vi "Query Chain.vi"(5 "Caller Enqueuer":refnum<class "Message Enqueuer.lvclass">, 7 "Close Connections (F)":bool, 8 "error in (no error)":errorcluster, 9 "Execute IL Action (T)":bool=TRUE, 11 "Interlock Chain":refnum<class "Interlock Chain.lvclass">) -> (0 "error out":errorcluster, 1 "Interlock?":bool, 2 "Interlock out":refnum<class "Interlock.lvclass">, 3 "Interlock Chain":refnum<class "Interlock Chain.lvclass">, 4 "Stop Self?":bool, 6 "IL Action":refnum<class "IL Action.lvclass">[](array[class]))   [LabVIEW 2015, in "Interlocks.lvlib" / "Interlock Chain.lvclass"]
uses:
  Interlock Chain/Interlock Chain.lvclass
  Interlock.lvclass
  IL Action/IL Action.lvclass
  <vilib>/ActorFramework/Message Enqueuer/Message Enqueuer.lvclass
  Interlock Chain/Interlock Chain.lvclass/Interlock Chain.ctl
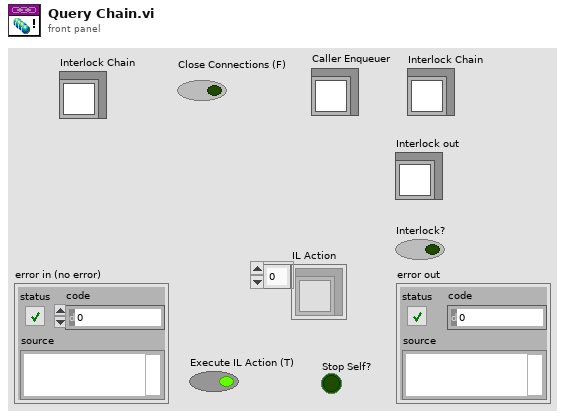
[diagram p1: front panel]
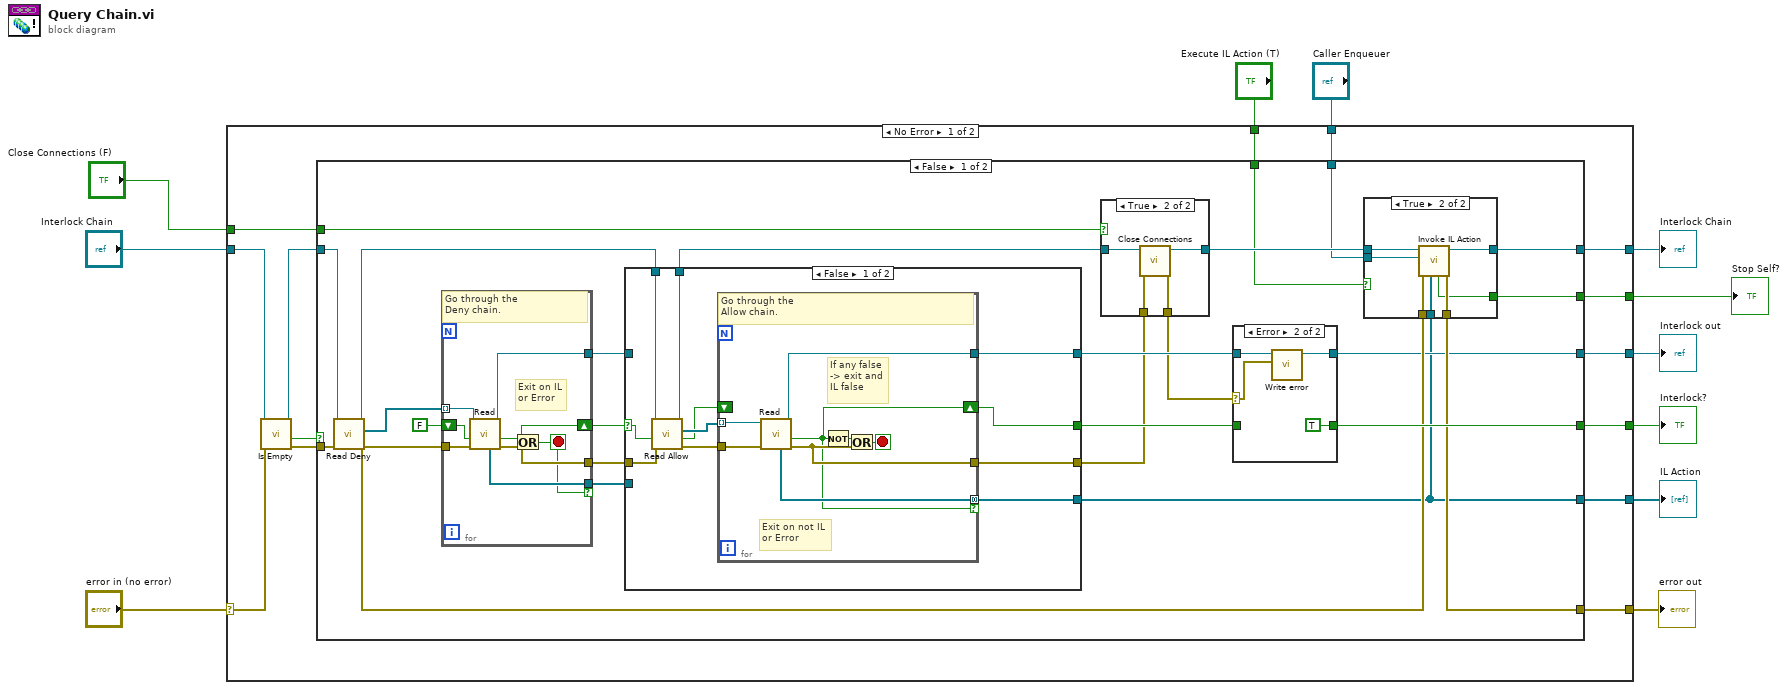
[diagram p0: block diagram]
diagram:
  n1 = case shown="No Error" "error in (no error)" {
    selector: "error in (no error)" -> [w15 w106]
    tunnel: "Interlock Chain" -> [w20 w107]
    tunnel: [w25 _] -> w11
    tunnel: [w24 _] -> w10
    tunnel: [w23 w107] -> w7
    tunnel: "Close Connections (F)" -> [w22 _]
    tunnel: [w17 _] -> w5
    tunnel: [w16 w106] -> w4
    tunnel: "Caller Enqueuer" -> [w14 _]
    tunnel: "Execute IL Action (T)" -> [w13 _]
    tunnel: [w12 _] -> w1
    frame No Error {
      n2 = call "Is Empty.vi"("error in (no error)"=w15, "Interlock Chain in"=w20) -> ("error out"=w21:errorcluster, "Is Empty?"=w18:bool, "Interlock Chain out"=w19:refnum<class "Interlock Chain.lvclass">)  [unwired: 7 in]
      n3 = case shown="False" w18 {
        tunnel: [w30 _] -> w25
        tunnel: [w41 _] -> w24
        tunnel: [w33 w105] -> w23
        tunnel: w22 -> [w39 _]
        tunnel: w21 -> [w38 w104]
        tunnel: w19 -> [w37 w105]
        tunnel: [w28 _] -> w17
        tunnel: [w31 w104] -> w16
        tunnel: w14 -> [w29 _]
        tunnel: w13 -> [w27 _]
        tunnel: [w26 _] -> w12
        frame False {
          n4 = call "Read Deny.vi"("error in (no error)"=w38, "Interlock Chain in"=w37) -> ("error out"=w32:errorcluster, "Deny"=w49:refnum<class "Interlock.lvclass">[], "Interlock Chain out"=w48:refnum<class "Interlock Chain.lvclass">)  [unwired: 7 in]
          n5 = for {
            shift-right: [w100] -> w43
            shift-left: FALSE ("Interlock out") -> [w102]
            tunnel: [w101] -> w45
            tunnel: w32 -> [w103]
            tunnel: [w98] -> w44
            tunnel: w49 -> [w99] mode=indexing
            tunnel: [w97] -> w36 if=w96
            stop <- w96 stop-if-true
            # "Exit on IL\nor Error"
            # "Go through the\nDeny chain."
            n6 = call-dynamic "Read.vi"("error in (no error)"=w103, 9:"Interlock in"=w102, 11:"Interlock in"=w99) -> ("error out"=w98:errorcluster, 1:"Interlock out"=w100:bool, 3:"Interlock out"=w101:refnum<class "Interlock.lvclass">, "IL Action"=w97:refnum<class "IL Action.lvclass">[])  [unwired: 4 in, 1 out]
            n7 = Or(x=w100, y=w98) -> (x .or. y?=w96:bool)
          }
          n8 = case shown="False" w43 {
            selector: w43 -> [w68 w89]
            tunnel: w48 -> [w76 w86]
            tunnel: [w75 w86] -> w47
            tunnel: [w70 w88] -> w46
            tunnel: w45 -> [_ w88]
            tunnel: [w69 w89] -> w42
            tunnel: [w72 w87] -> w40
            tunnel: w44 -> [w71 w87]
            tunnel: w36 -> [_ w85]
            tunnel: [w66 w85] -> w28
            frame False {
              n9 = call "Read Allow.vi"("error in (no error)"=w71, "Interlock in (False)"=w68, "Interlock Chain in"=w76) -> ("error out"=w74:errorcluster, "Interlock out"=w67:bool, "Allow"=w73:refnum<class "Interlock.lvclass">[], "Interlock Chain out"=w75:refnum<class "Interlock Chain.lvclass">)  [unwired: 5 in]
              n10 = for {
                tunnel: w74 -> [w84]
                tunnel: [w82] -> w72
                tunnel: w73 -> [w83] mode=indexing
                tunnel: [w81] -> w70
                shift-right: [w77] -> w69
                shift-left: w67 -> [_]
                tunnel: [w80] -> w66 mode=concatenating if=w77
                stop <- w79 stop-if-true
                # "If any false\n-> exit and\nIL false"
                # "Exit on not IL\nor Error"
                # "Go through the\nAllow chain."
                n11 = call-dynamic "Read.vi"("error in (no error)"=w84, "Interlock in"=w83) -> ("error out"=w82:errorcluster, 1:"Interlock out"=w77:bool, 3:"Interlock out"=w81:refnum<class "Interlock.lvclass">, "IL Action"=w80:refnum<class "IL Action.lvclass">[])  [unwired: 5 in, 1 out]
                n12 = Not(x=w77) -> (.not. x?=w78:bool)
                n13 = Or(x=w78, y=w82) -> (x .or. y?=w79:bool)
              }
            }
            frame True {
            }
          }
          n14 = case shown="True" w39 {
            tunnel: w47 -> [w61 w65]
            tunnel: [w61 w64] -> w34
            tunnel: w40 -> [w60 w63]
            tunnel: [w60 w62] -> w35
            frame False {
            }
            frame True {
              n15 = call "Close Connections.vi"("error in (no error)"=w63, "Interlock Chain in"=w65) -> ("error out"=w62:errorcluster, "Interlock Chain out"=w64:refnum<class "Interlock Chain.lvclass">)  [unwired: 8 in]
            }
          }
          n16 = case shown="Error" w35 {
            selector: w35 -> [_ w93]
            tunnel: w46 -> [w91 w95]
            tunnel: [w91 w94] -> w30
            tunnel: w42 -> [w90 _]
            tunnel: [w90 TRUE ("Interlock out")] -> w41
            frame No Error {
            }
            frame Error {
              n17 = call "Write error.vi"("error"=w93, "Interlock in"=w95) -> ("Interlock out"=w94:refnum<class "Interlock.lvclass">)  [unwired: 9 in]
            }
          }
          n18 = case shown="True" w27 {
            tunnel: w34 -> [w51 w59]
            tunnel: [w51 w58] -> w33
            tunnel: w32 -> [w52 w57]
            tunnel: [w52 w56] -> w31
            tunnel: w29 -> [_ w54]
            tunnel: w28 -> [_ w55]
            tunnel: [_ w53] -> w26
            frame False {
            }
            frame True {
              n19 = call "Invoke IL Action.vi"("IL Action"=w55, "error in (no error)"=w57, "Caller Enqueuer"=w54, "Interlock Chain in"=w59) -> ("error out"=w56:errorcluster, "Interlock Chain out"=w58:refnum<class "Interlock Chain.lvclass">, "Stop Self?"=w53:bool)  [unwired: 5 in]
            }
          }
        }
        frame True {
          # "The chain is empty, nothing to do here"
        }
      }
    }
    frame Error {
    }
  }
  "error out" <- w4
  "Interlock out" <- w11
  "Interlock?" <- w10
  "Interlock Chain" <- w7
  "IL Action" <- w5
  "Stop Self?" <- w1
